vi "Calc.vi"(6 "ScanTableSize":i32[](array[numeric]), 8 "error in (no error)":errorcluster caption="entrée d'erreur (pas d'erreur)", 10 "AllPointIndex":i32, 11 "InstrClassIn":refnum<class "Calculations.lvclass"> caption="DNL_LabVIEW Object in") -> (0 "error out":errorcluster caption="sortie d'erreur", 2 "MeasDatOut":dbl[](array[numeric]), 3 "InstrClassOut":refnum<class "Calculations.lvclass"> caption="DNL_LabVIEW Object out")   [LabVIEW 2019, in "Calculations.lvclass"]
uses:
  Calculations.lvclass
  Calculations.lvclass/Calculations.ctl
  <vilib>/Analysis/baseanly.llb/Mean (DBL).vi
  <vilib>/Analysis/NI_AALBase.lvlib
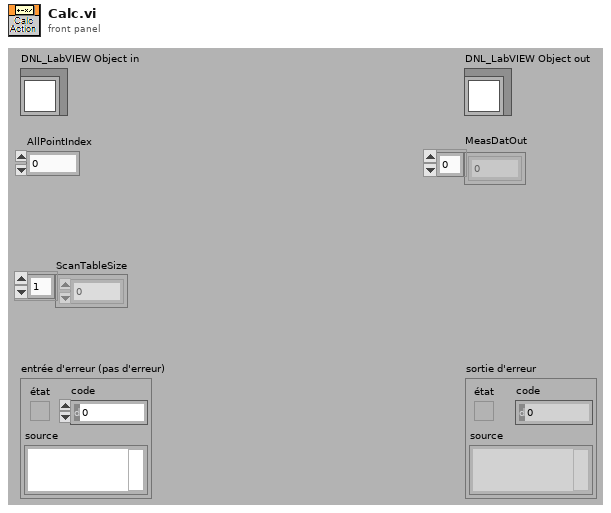
[diagram p1: front panel]
types:
  T1 = typedef "Calculations.lvclass/DefaultDev_Func.ctl" = enum16{"Multi Scan Average", "Running Average", "Summ"}
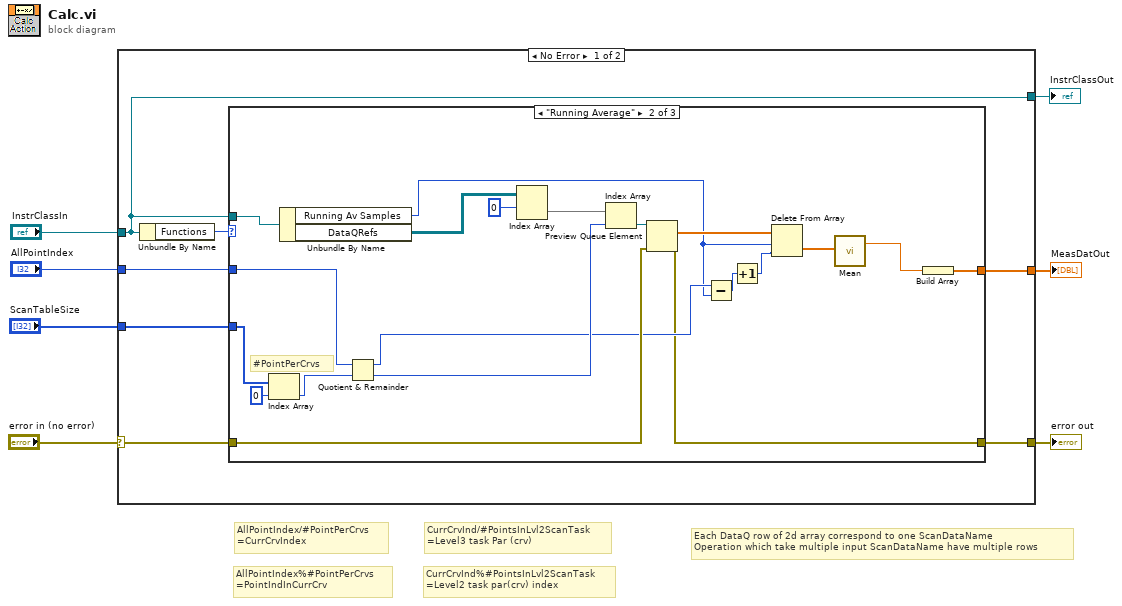
[diagram p0: block diagram]
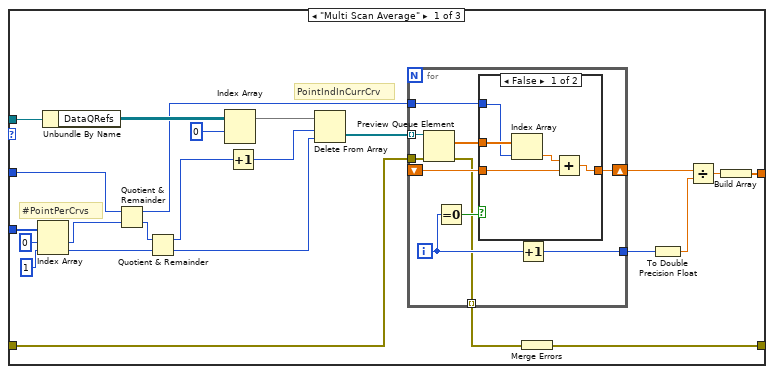
[diagram p2: hidden frame]
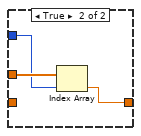
[diagram p3: hidden frame]
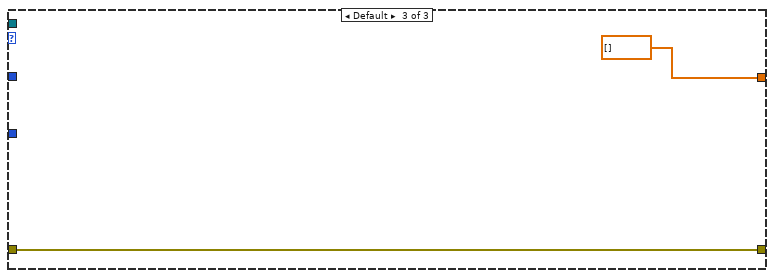
[diagram p4: hidden frame]
diagram:
  # "Each DataQ row of 2d array correspond to one ScanDataName\nOperation which take multiple input ScanDataName have multiple rows"
  # "CurrCrvInd%#PointsInLvl2ScanTask\n=Level2 task par(crv) index"
  # "AllPointIndex%#PointPerCrvs\n=PointIndInCurrCrv"
  # "CurrCrvInd/#PointsInLvl2ScanTask\n=Level3 task Par (crv)"
  # "AllPointIndex/#PointPerCrvs\n=CurrCrvIndex"
  n1 = case shown="No Error" "error in (no error)" {
    selector: "error in (no error)" -> [w10 w79]
    tunnel: "InstrClassIn" -> [w9 w80]
    tunnel: [w9 w80] -> w5
    tunnel: "AllPointIndex" -> [w14 _]
    tunnel: [w13 w79] -> w3
    tunnel: [w12 _] -> w2
    tunnel: "ScanTableSize" -> [w8 _]
    frame No Error {
      n2 = Unbundle By Name(w9) -> ("Functions"=w11:T1)
      n3 = case shown="\"Running Average\"" w11 {
        tunnel: w14 -> [w28 w70 _]
        tunnel: [w18 w57 w77] -> w13
        tunnel: [w26 w58 dbl[] [] ("Outputs")] -> w12
        tunnel: w10 -> [w20 w66 w77]
        tunnel: w9 -> [w38 w76 _]
        tunnel: w8 -> [w36 w71 _]
        frame "Multi Scan Average" {
          # "PointIndInCurrCrv"
          # "#PointPerCrvs"
          n4 = Index Array(array=w36, index #1=0 ("index"), index #2=1 ("index")) -> (element #1=w29:i32, element #2=w23:i32)
          n5 = Unbundle By Name(w38) -> ("DataQRefs"=w37:refnum<queue>[][])
          n6 = Quotient & Remainder(x=w28, y=w29) -> (x-y*floor(x/y)=w17:i32, floor(x/y)=w27:i32)
          n7 = Quotient & Remainder(x=w27, y=w23) -> (x-y*floor(x/y)=w25:i32, floor(x/y)=w22:i32)
          n8 = Index Array(array=w37, index (row)=0) -> (element=w34:refnum<queue>[])  [unwired: 1 in]
          n9 = Increment(x=w25) -> (x+1=w24:i32)
          n10 = Delete From Array(array=w34, length=w24, index=w22) -> (deleted portion=w32:refnum<queue>[])  [unwired: 1 out]
          n11 = for {
            tunnel: w32 -> [w48] mode=indexing
            tunnel: [w42] -> w31
            shift-right: [w46] -> w16
            shift-left: _ -> [w45]
            tunnel: w20 -> [w41]
            tunnel: [w40] -> w19 mode=indexing
            tunnel: w17 -> [w39]
            i -> [w43]
            n12 = Preview Queue Element(queue=w48, error in (no error)=w41) -> (element=w47:dbl[], error out=w40:errorcluster)  [unwired: 1 in, 2 out]
            n13 = Equal To 0?(x=w43) -> (x = 0?=w44:bool)
            n14 = case shown="False" w44 {
              tunnel: w47 -> [w52 w56]
              tunnel: w45 -> [w49 _]
              tunnel: [w53 w54] -> w46
              tunnel: w39 -> [w50 w55]
              frame False {
                n15 = Index Array(array=w52, index=w50) -> (element=w51:dbl)
                n16 = Add(x=w51, y=w49) -> (x+y=w53:dbl)
              }
              frame True {
                n17 = Index Array(array=w56, index=w55) -> (element=w54:dbl)
              }
            }
            n18 = Increment(x=w43) -> (x+1=w42:i32)
          }
          n19 = Merge Errors(w19) -> (w18:errorcluster)
          n20 = To Double Precision Float(number=w31) -> (double precision float=w30:dbl)
          n21 = Divide(x=w16, y=w30) -> (x/y=w15:dbl)
          n22 = Build Array(w15) -> (w26:dbl[])
        }
        frame "Running Average" {
          # "#PointPerCrvs"
          n23 = Index Array(array=w71, index=0) -> (element=w72:i32)
          n24 = Unbundle By Name(w76) -> ("Running Av Samples"=w61:i32, "DataQRefs"=w74:refnum<queue>[][])
          n25 = Quotient & Remainder(x=w70, y=w72) -> (x-y*floor(x/y)=w62:i32, floor(x/y)=w67:i32)
          n26 = Index Array(array=w74, index (row)=0) -> (element=w69:refnum<queue>[])  [unwired: 1 in]
          n27 = Index Array(array=w69, index=w67) -> (element=w68:refnum<queue>)
          n28 = Preview Queue Element(queue=w68, error in (no error)=w66) -> (element=w65:dbl[], error out=w57:errorcluster)  [unwired: 1 in, 2 out]
          n29 = Subtract(x=w62, y=w61) -> (x-y=w64:i32)
          n30 = Increment(x=w64) -> (x+1=w63:i32)
          n31 = Delete From Array(array=w65, length=w61, index=w63) -> (deleted portion=w60:dbl[])  [unwired: 1 out]
          n32 = call-poly <vilib>:"Mean.vi"("X"=w60) -> ("mean"=w59:dbl)  [unwired: 1 out]
          n33 = Build Array(w59) -> (w58:dbl[])
        }
        frame Default {
        }
      }
    }
    frame Error {
    }
  }
  "error out" <- w3
  "InstrClassOut" <- w5
  "MeasDatOut" <- w2
